vi "winFormsSubVI searchText.vi"(8 "error in (no error)":errorcluster, 10 "searchString":string, 11 "scintillaRefNum in":refnum<k24>) -> (0 "error out":errorcluster, 3 "scintillaRefNum out":refnum<k24>)   [LabVIEW 2018]
uses:
  C:/ATI_MS_InstrumentControl/dll/ScintillaNET.dll
  dll/ScintillaNET.dll
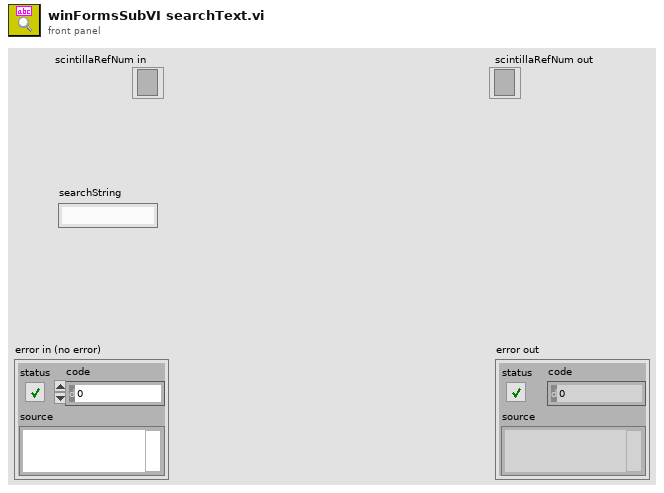
[diagram p1: front panel]
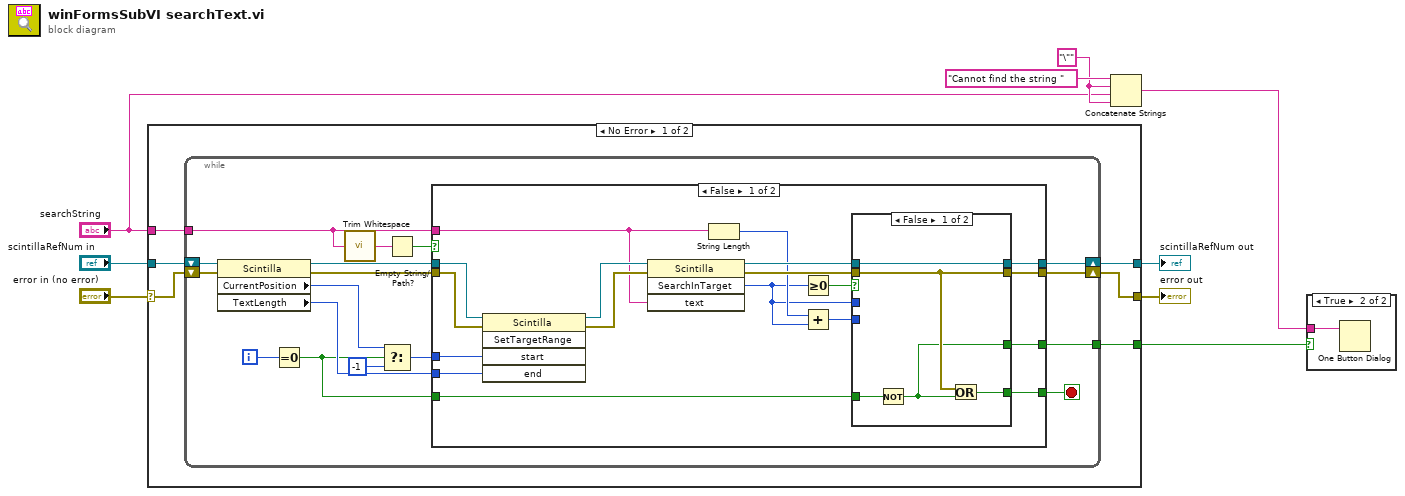
[diagram p0: block diagram]
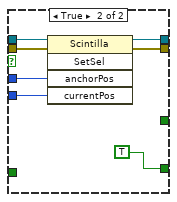
[diagram p3: hidden frame]
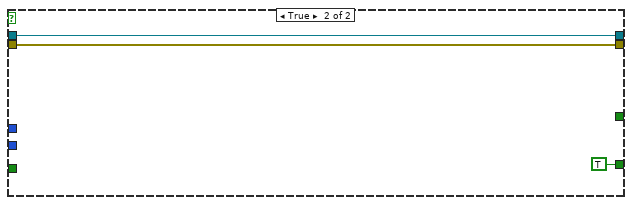
[diagram p4: hidden frame]
diagram:
  w3 = "\""
  n1 = case shown="No Error" "error in (no error)" {
    selector: "error in (no error)" -> [w13 w67]
    tunnel: "searchString" -> [w15 _]
    tunnel: "scintillaRefNum in" -> [w14 w66]
    tunnel: [w12 w67] -> w7
    tunnel: [w11 w66] -> w6
    tunnel: [w10 _] -> w5
    frame No Error {
      n2 = while {
        tunnel: w15 -> [w20]
        shift-right: [w26] -> w11
        shift-left: w14 -> [w24]
        shift-right: [w25] -> w12
        shift-left: w13 -> [w23]
        tunnel: [w22] -> w10
        i -> [w32]
        stop <- w27 stop-if-true
        n3 = property class="Scintilla"(reference=w24, error in=w23) -> (reference out=w17:refnum<k24>, error out=w16:errorcluster, "CurrentPosition"=w31:i32, "TextLength"=w28:i32)
        n4 = Equal To 0?(x=w32) -> (x = 0?=w21:bool)
        n5 = call <vilib>:"Trim Whitespace.vi"("string"=w20) -> ("trimmed string"=w18:string)  [unwired: 1 in]
        n6 = Select(t=w31, s=w21, f=-1) -> (s? t:f=w29:i32)
        n7 = Empty String/Path?(string/path=w18) -> (empty?=w19:bool)
        n8 = case shown="False" w19 {
          tunnel: w17 -> [w50 w65]
          tunnel: w16 -> [w49 w64]
          tunnel: w29 -> [w48 _]
          tunnel: w28 -> [w47 _]
          tunnel: [w38 TRUE] -> w27
          tunnel: [w37 w65] -> w26
          tunnel: [w36 w64] -> w25
          tunnel: [w35 _] -> w22
          tunnel: w21 -> [w34 _]
          tunnel: w20 -> [w33 _]
          frame False {
            n9 = invoke class="Scintilla" method="SetTargetRange"(reference=w50, error in=w49, "start"=w48, "end"=w47) -> (reference out=w46:refnum<k24>, error out=w45:errorcluster)  [unwired: 1 in, 3 out]
            n10 = invoke class="Scintilla" method="SearchInTarget"(reference=w46, error in=w45, "text"=w33) -> (reference out=w44:refnum<k24>, error out=w43:errorcluster, "SearchInTarget"=w40:i32)  [unwired: 1 in, 1 out]
            n11 = String Length(string=w33) -> (length=w41:i32)
            n12 = Greater Or Equal To 0?(x=w40) -> (x >= 0?=w42:bool)
            n13 = Add(x=w41, y=w40) -> (x+y=w39:i32)
            n14 = case shown="False" w42 {
              tunnel: w44 -> [w55 w62]
              tunnel: w43 -> [w53 w61]
              tunnel: w39 -> [_ w60]
              tunnel: [w53 w59] -> w36
              tunnel: w40 -> [_ w58]
              tunnel: [w55 w57] -> w37
              tunnel: w34 -> [w54 _]
              tunnel: [w52 TRUE] -> w38
              tunnel: [w51 _] -> w35
              frame False {
                n15 = Not(x=w54) -> (.not. x?=w51:bool)
                n16 = Or(x=w53, y=w51) -> (x .or. y?=w52:bool)
              }
              frame True {
                n17 = invoke class="Scintilla" method="SetSel"(reference=w62, error in=w61, "anchorPos"=w58, "currentPos"=w60) -> (reference out=w57:refnum<k24>, error out=w59:errorcluster)  [unwired: 1 in, 3 out]
              }
            }
          }
          frame True {
          }
        }
      }
    }
    frame Error {
    }
  }
  "scintillaRefNum out" <- w6
  "error out" <- w7
  n18 = Concatenate Strings("Cannot find the string ", w3, "searchString", w3) -> (w2:string)
  n19 = case shown="True" w5 {
    tunnel: w2 -> [_ w68]
    frame False {
    }
    frame True {
      n20 = One Button Dialog(message=w68) -> ()  [unwired: 1 in, 1 out]
    }
  }
